vi "Current Sense_t.vi"() -> ()   [LabVIEW 2022 SP3]
uses:
  <vilib>/DAQmx/write.llb/DAQmx Write (Analog 1D DBL 1Chan NSamp).vi
  <vilib>/DAQmx/read.llb/DAQmx Read (Analog Wfm 1Chan NSamp).vi
  <vilib>/DAQmx/miscellaneous.llb/DAQmx Fill In Error Info.vi
panel:
  out "error out":errorcluster
  in  "error in":errorcluster
  out "data":dbl format="%0.2f"
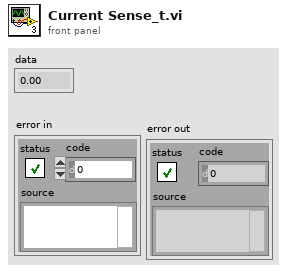
[diagram p1: front panel]
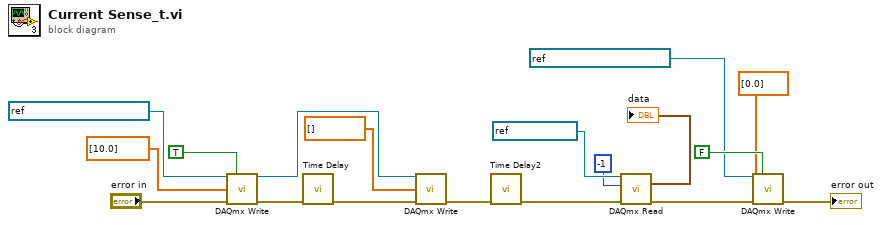
[diagram p0: block diagram]
diagram:
  n1 = call-poly <vilib>:"DAQmx Write.vi"("task/channels in"=refnum<k21> "Current Sensors_BON", "auto start"=TRUE, "data"=dbl[] [10.0], "error in"="error in") -> ("task out"=w7:refnum<k21>, "error out"=w17:errorcluster)  [unwired: 9 in, 1 out]
  n2 = call "Time Delay"("error in (no error)"=w17) -> ("error out"=w8:errorcluster)  [unwired: 10 in]
  n3 = call-poly <vilib>:"DAQmx Write.vi"("task/channels in"=w7, "data"=dbl[] [], "error in"=w8) -> ("error out"=w5:errorcluster)  [unwired: 10 in, 2 out]
  n4 = call "Time Delay2"("error in (no error)"=w5) -> ("error out"=w4:errorcluster)  [unwired: 10 in]
  n5 = call-poly <vilib>:"DAQmx Read.vi"("task/channels in"=refnum<k21> "ISENSE_C+", "number of samples per channel"=-1, "error in"=w4) -> ("data"=→"data":waveform(dbl), "error out"=w11:errorcluster)  [unwired: 10 in, 1 out]
  n6 = call-poly <vilib>:"DAQmx Write.vi"("task/channels in"=refnum<k21> "Current Sensors_BON", "auto start"=FALSE, "data"=dbl[] [0.0], "error in"=w11) -> ("error out"=→"error out":errorcluster)  [unwired: 9 in, 2 out]
